vi "IntakeExecute.vi"(8 "error in (no error)":errorcluster) -> (0 "error out":errorcluster)   [LabVIEW 2023]
uses:
  <vilib>/Rock Robotics/WPI/ThirdParty/REV Robotics/REVLib/Typedef/Spark MAX Control Type.ctl
  <vilib>/Rock Robotics/WPI/ThirdParty/JAS_Junk/TrajLib/Timer_New.vi
  <vilib>/Utility/semaphor.llb/Obtain Semaphore Reference.vi
  <vilib>/Rock Robotics/WPI/ThirdParty/JAS_Junk/TrajLib/Timer_Reset.vi
  <vilib>/Rock Robotics/WPI/ThirdParty/JAS_Junk/TrajLib/Timer_Start.vi
  <vilib>/Rock Robotics/WPI/ThirdParty/JAS_Junk/TrajLib/Timer_Stop.vi
  <vilib>/Rock Robotics/WPI/ThirdParty/JAS_Junk/TrajLib/Timer_HasPeriodPassedOnce.vi
  <vilib>/Rock Robotics/WPI/ThirdParty/JAS_Junk/TrajLib/Trajectory_Library.lvlib
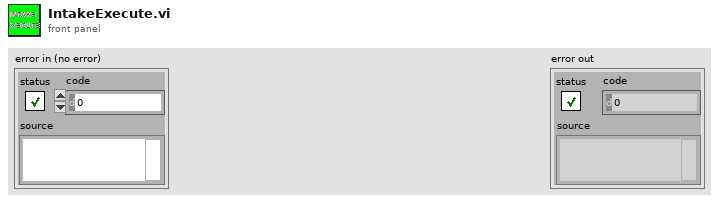
[diagram p1: front panel]
types:
  T1 = typedef "Spark MAX Control Type.ctl" = enum16{"Percent VBus", "Voltage", "Velocity", "Position", "Smart Motion", "Current", "Smart Velocity", "MAXMotion Position", "MAXMotion Velocity"}
  T2 = typedef "WPI_MotorControlDeviceRef.ctl" = cluster{"DeviceStatus":errorcluster, "Type":T3, "PWM":cluster{"PWM Channel":T4, "DeadBand":T5}, "CAN":cluster{"Device Number":u8, "SetOutput VI Ref":variant, "GetOutput VI Ref":variant, "Enable VI Ref":variant, "Disable VI Ref":variant, "Data":variant}, "Invert":bool, "DIO PWM":cluster{"PWM \"Enable\" Channel":T4, "DIOChannel":T6, "PWM Rate":dbl}}
  T3 = typedef "WPI_MotorControlType.ctl" = enum16{"PWM", "CAN", "DIO PWM"}
  T4 = typedef "FPGA_DIOPWMChannel.ctl" = enum8{"PWM 0", "PWM 1", "PWM 2", "PWM 3", "PWM 4", "PWM 5", "PWM 6", "PWM 7", "PWM 8", "PWM 9", "PWM MXP 0", "PWM MXP 1", "PWM MXP 2", "PWM MXP 3", "PWM MXP 4", "PWM MXP 5", "PWM MXP 6", "PWM MXP 7", "PWM MXP 8", "PWM MXP 9", "Invalid"}
  T5 = typedef "WPI_PWMDeadband.ctl" = cluster{"Name":string, "maxPositivePwm":i32, "minPositivePwm":i32, "centerPwm":i32, "maxNegativePwm":i32, "minNegativePwm":i32, "angularRange":u16}
  T6 = typedef "FPGA_DIOChannel.ctl" = enum8{"DIO 0", "DIO 1", "DIO 2", "DIO 3", "DIO 4", "DIO 5", "DIO 6", "DIO 7", "DIO 8", "DIO 9", "DIO MXP 0", "DIO MXP 1", "DIO MXP 2", "DIO MXP 3", "DIO MXP 4", "DIO MXP 5", "DIO MXP 6", "DIO MXP 7", "DIO MXP 8", "DIO MXP 9", "DIO MXP 10", "DIO MXP 11", "DIO MXP 12", "DIO MXP 13", "DIO MXP 14", "DIO MXP 15", "SPI Port CS1", "SPI Port CS2", "SPI Port CS3", "SPI Port MISO", "SPI Port MOSI", "Invalid"}
  T7 = typedef "WPI_SwitchDevRef.ctl" = cluster{"DevStatus":errorcluster, "DIO Channel":T6, "CntIndex":T8, "Normally Closed":bool}
  T8 = typedef "FPGA_CounterCtrSystemIndex.ctl" = enum8{"Ctr 0", "Ctr 1", "Ctr 2", "Ctr 3", "Ctr 4", "Ctr 5", "Ctr 6", "Ctr 7", "Invalid"}
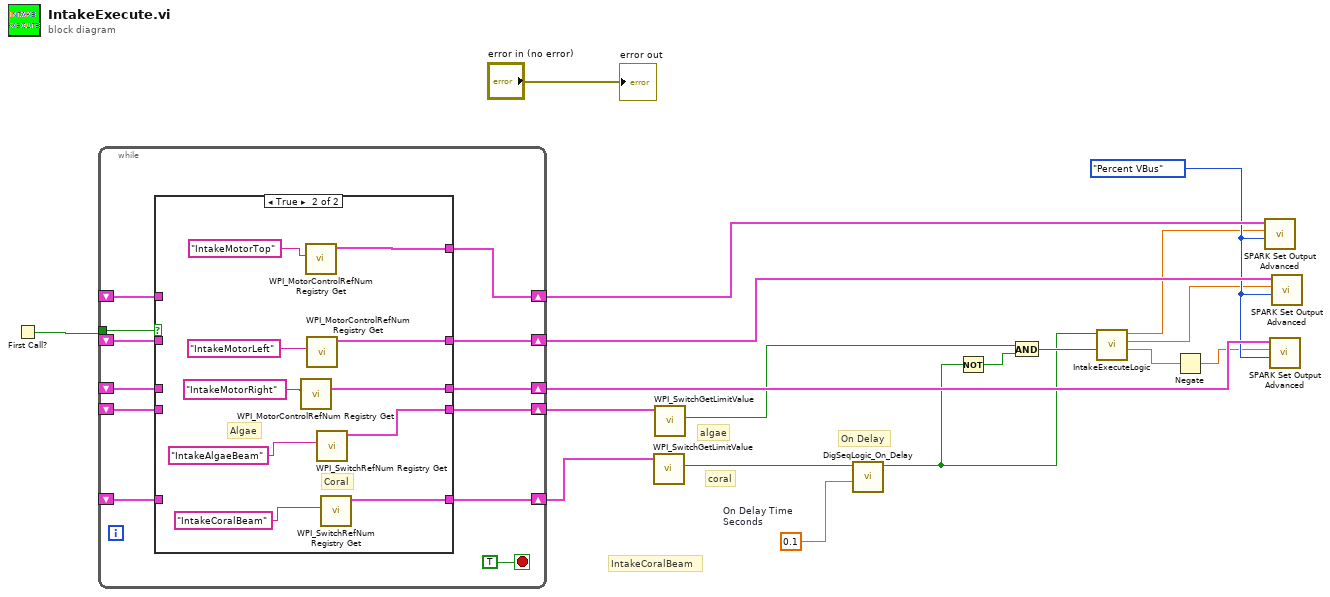
[diagram p0: block diagram]
diagram:
  w6 = 0.1  # On Delay Time Seconds
  w12 = Spark_MAX_Control_Type."Percent VBus" ("Control Mode")
  # "On Delay"
  # "algae"
  # "coral"
  # "IntakeCoralBeam"
  n1 = First Call?() -> (First Call?: T/F=w17:bool)
  n2 = while {
    tunnel: w17 -> [w29]
    shift-right: [w30] -> w14
    shift-left: _ -> [w28]
    shift-right: [w26] -> w15
    shift-left: _ -> [w25]
    shift-right: [w24] -> w13
    shift-left: _ -> [w23]
    shift-right: [w22] -> w16
    shift-left: _ -> [w21]
    shift-right: [w20] -> w9
    shift-left: _ -> [w19]
    stop <- TRUE stop-if-true
    n3 = case shown="True" w29 {
      tunnel: [w35 w43] -> w30
      tunnel: w28 -> [w35 _]
      tunnel: [w34 w42] -> w26
      tunnel: w25 -> [w34 _]
      tunnel: [w33 w41] -> w24
      tunnel: w23 -> [w33 _]
      tunnel: [w32 w39] -> w22
      tunnel: w21 -> [w32 _]
      tunnel: [w31 w37] -> w20
      tunnel: w19 -> [w31 _]
      frame False {
      }
      frame True {
        # "Algae"
        # "Coral"
        n4 = call <vilib>:"WPI_MotorControlRefNum Registry Get.vi"("refnum name"="IntakeMotorRight") -> ("MotorControlDevRef"=w43:T2)  [unwired: 9 in, 1 out]
        n5 = call <vilib>:"WPI_MotorControlRefNum Registry Get.vi"("refnum name"="IntakeMotorTop") -> ("MotorControlDevRef"=w41:T2)  [unwired: 9 in, 1 out]
        n6 = call <vilib>:"WPI_MotorControlRefNum Registry Get.vi"("refnum name"="IntakeMotorLeft") -> ("MotorControlDevRef"=w42:T2)  [unwired: 9 in, 1 out]
        n7 = call <vilib>:"WPI_SwitchRefNum Registry Get.vi"("refnum name"="IntakeAlgaeBeam") -> ("SwitchDevRef"=w39:T7)  [unwired: 9 in, 1 out]
        n8 = call <vilib>:"WPI_SwitchRefNum Registry Get.vi"("refnum name"="IntakeCoralBeam") -> ("SwitchDevRef"=w37:T7)  [unwired: 9 in, 1 out]
      }
    }
  }
  n9 = call <vilib>:"WPI_SwitchGetLimitValue.vi"("SwitchDevRef"=w9) -> ("Switch Pressed"=w5:bool)  [unwired: 8 in, 2 out]
  n10 = call <vilib>:"WPI_SwitchGetLimitValue.vi"("SwitchDevRef"=w16) -> ("Switch Pressed"=w4:bool)  [unwired: 8 in, 2 out]
  n11 = call <vilib>:"DigSeqLogic_On_Delay.vi"("Delay"=w6, "Input"=w5) -> ("Output"=w1:bool)  [unwired: 8 in, 1 out]
  n12 = Not(x=w1) -> (.not. x?=w2:bool)
  n13 = And(x=w4, y=w2) -> (x .and. y?=w3:bool)
  n14 = call "IntakeExecuteLogic.vi"("HaveAlgaeSensor"=w3, "HaveCoralSensor"=w1) -> ("MotorDemandRight"=w8:dbl, "MotorDemandLeft"=w11:dbl, "MotorDemandTop"=w10:dbl)  [unwired: 6 in, 1 out]
  n15 = Negate(x=w8) -> (-x=w7:dbl)
  n16 = call <vilib>:"SPARK Set Output Advanced.vi"("Control Mode"=w12, "Setpoint"=w10, "MotorControlDevRef"=w13) -> ()  [unwired: 7 in, 2 out]
  n17 = call <vilib>:"SPARK Set Output Advanced.vi"("Control Mode"=w12, "Setpoint"=w7, "MotorControlDevRef"=w14) -> ()  [unwired: 7 in, 2 out]
  n18 = call <vilib>:"SPARK Set Output Advanced.vi"("Control Mode"=w12, "Setpoint"=w11, "MotorControlDevRef"=w15) -> ()  [unwired: 7 in, 2 out]
  "error out" <- "error in (no error)"
